vi "Get Method Resource.vi"(7 "LabVIEW Web Service Request":refnum<class "Web Request.lvclass">, 8 "start":dbl, 9 "getdata":dbl, 10 "stop":dbl, 11 "save_file":dbl) -> (2 "Chassis Temperature":dbl, 3 "value":string)   [LabVIEW 2020]
uses:
  <vilib>/wsapi/Web Request.lvclass
panel:
  # "Use the Web Service Request input terminal to call the VIs on the Web Services palette. Do not remove it from the connector pane unless you don't need access to the palette."
  # "Each additional control wired to the connector pane will be available as an input in the URL. To include an indicator in terminal-mode output (the default setting), it must also be wired to the connector pane."
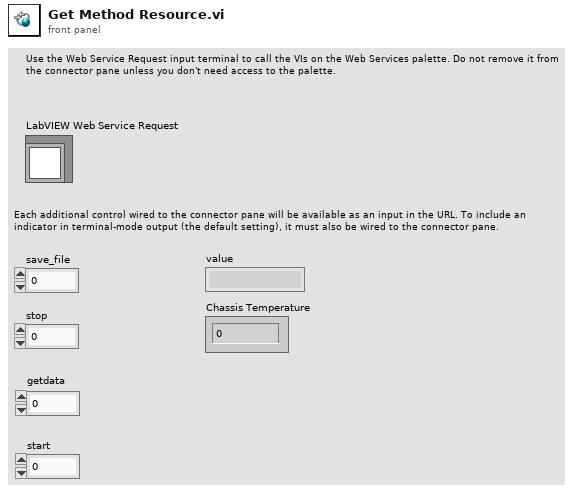
[diagram p1: front panel]
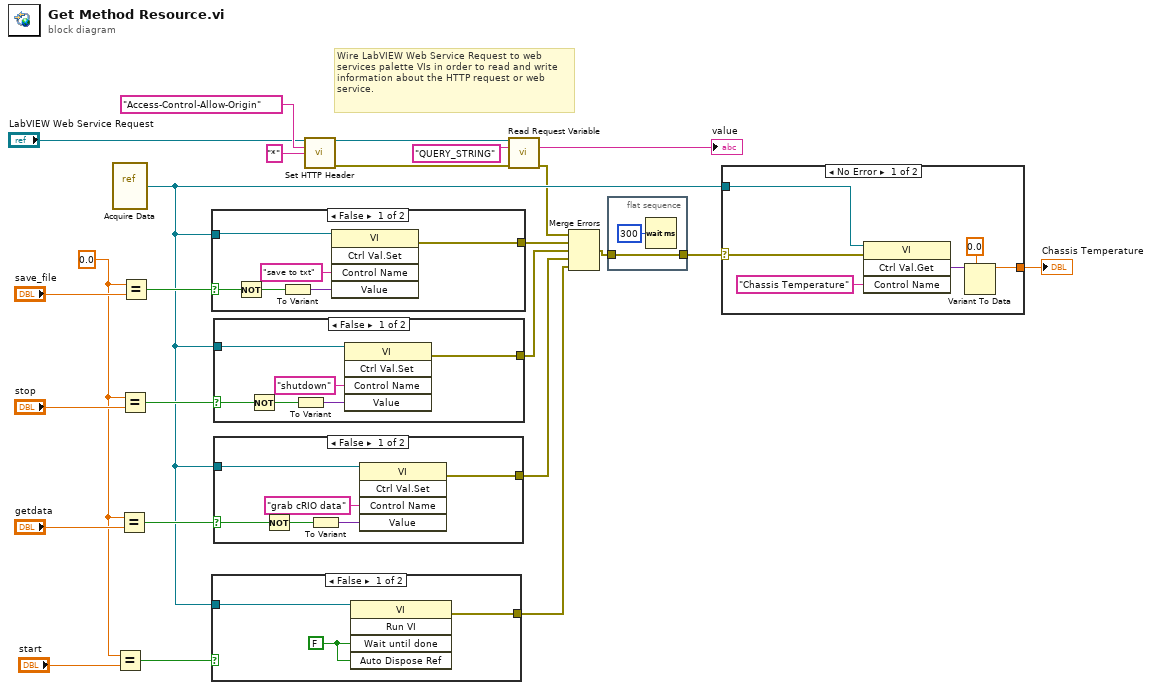
[diagram p0: block diagram]
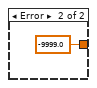
[diagram p2: hidden frame]
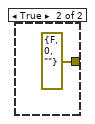
[diagram p3: hidden frame]
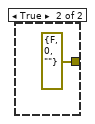
[diagram p4: hidden frame]
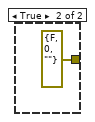
[diagram p5: hidden frame]
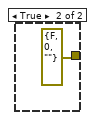
[diagram p6: hidden frame]
diagram:
  w11 = 0.0 ("x")
  # "Wire LabVIEW Web Service Request to web services palette VIs in order to read and write information about the HTTP request or web service."
  n1 = vi-ref "Acquire Data.vi"() -> (w13:refnum<vi>)
  n2 = Equal?(x=w11, y="start") -> (x = y?=w9:bool)
  n3 = Equal?(x=w11, y="getdata") -> (x = y?=w19:bool)
  n4 = Equal?(x=w11, y="stop") -> (x = y?=w18:bool)
  n5 = Equal?(x=w11, y="save_file") -> (x = y?=w20:bool)
  n6 = case shown="False" w20 {
    selector: w20 -> [w30 _]
    tunnel: w13 -> [w31 _]
    tunnel: [w26 errorcluster {"status"=FALSE, "code"=0, "source"=""} ("error out")] -> w15
    frame False {
      n7 = Not(x=w30) -> (.not. x?=w28:bool)
      n8 = To Variant(anything=w28) -> (Variant=w29:variant)
      n9 = invoke class="VI" method="Ctrl Val.Set"(reference=w31, "Control Name"="save to txt", "Value"=w29) -> (error out=w26:errorcluster)  [unwired: 2 in, 4 out]
    }
    frame True {
    }
  }
  n10 = case shown="False" w9 {
    tunnel: w13 -> [w35 _]
    tunnel: [w34 errorcluster {"status"=FALSE, "code"=0, "source"=""} ("error out")] -> w12
    frame False {
      w33 = FALSE ("Wait Until Done")
      n11 = invoke class="VI" method="Run VI"(reference=w35, "Wait until done"=w33, "Auto Dispose Ref"=w33) -> (error out=w34:errorcluster)  [unwired: 2 in, 4 out]
    }
    frame True {
    }
  }
  n12 = case shown="False" w18 {
    selector: w18 -> [w39 _]
    tunnel: w13 -> [w38 _]
    tunnel: [w37 errorcluster {"status"=FALSE, "code"=0, "source"=""} ("error out")] -> w16
    frame False {
      n13 = Not(x=w39) -> (.not. x?=w41:bool)
      n14 = To Variant(anything=w41) -> (Variant=w40:variant)
      n15 = invoke class="VI" method="Ctrl Val.Set"(reference=w38, "Control Name"="shutdown", "Value"=w40) -> (error out=w37:errorcluster)  [unwired: 2 in, 4 out]
    }
    frame True {
    }
  }
  n16 = case shown="False" w19 {
    selector: w19 -> [w46 _]
    tunnel: w13 -> [w45 _]
    tunnel: [w44 errorcluster {"status"=FALSE, "code"=0, "source"=""} ("error out")] -> w17
    frame False {
      n17 = Not(x=w46) -> (.not. x?=w48:bool)
      n18 = To Variant(anything=w48) -> (Variant=w49:variant)
      n19 = invoke class="VI" method="Ctrl Val.Set"(reference=w45, "Control Name"="grab cRIO data", "Value"=w49) -> (error out=w44:errorcluster)  [unwired: 2 in, 4 out]
    }
    frame True {
    }
  }
  n20 = call <vilib>:"Set HTTP Header.vi"("LabVIEW Web Service Request"="LabVIEW Web Service Request", "header"="Access-Control-Allow-Origin", "header value"="*") -> ("LabVIEW Web Service Request out"=w8:refnum<class "Web Request.lvclass">, "error out"=w7:errorcluster)  [unwired: 11 in]
  n21 = call <vilib>:"Read Request Variable.vi"("LabVIEW Web Service Request"=w8, "variable name"="QUERY_STRING", "error in (no error)"=w7) -> ("value"=→"value":string, "error out"=w6:errorcluster)  [unwired: 10 in, 1 out]
  n22 = Merge Errors(w6, w15, w16, w17, w12) -> (w14:errorcluster)
  n23 = flat-sequence {
    tunnel: w14 -> [w51]
    tunnel: [w51] -> w2
    frame #0 {
      n24 = Wait (ms)(milliseconds to wait=u32 300) -> ()  [unwired: 1 out]
    }
  }
  n25 = case shown="No Error" w2 {
    selector: w2 -> [w54 _]
    tunnel: w13 -> [w55 _]
    tunnel: [w53 -9999.0] -> w1
    frame No Error {
      n26 = invoke class="VI" method="Ctrl Val.Get"(reference=w55, error in=w54, "Control Name"="Chassis Temperature") -> ("Get Control Value Variant"=w57:variant)  [unwired: 1 in, 3 out]
      n27 = Variant To Data(type=0.0, Variant=w57) -> (data=w53:dbl)  [unwired: 1 in, 1 out]
    }
    frame Error {
    }
  }
  "Chassis Temperature" <- w1
